vi "CreateChannel.vi"(6 "Units":string, 8 "error in (no error)":errorcluster, 9 "ChannelName":string, 10 "ChannelID":string, 11 "FPGA reference":refnum<k20>) -> (0 "error out":errorcluster, 3 "9770 API out":refnum<class "9770 API.lvclass">)   [LabVIEW 2017, in "9770 API.lvclass"]
uses:
  <vilib>/addons/InsightCM/Devices/Shared/Emsa/Emsa9770API/9770 API.lvclass
  <vilib>/addons/InsightCM/Devices/Shared/Emsa/Emsa9770API/controls/FPGATypeDef.ctl
  <vilib>/addons/InsightCM/Devices/Shared/Emsa/Emsa9770API/9770 API.lvclass/9770 API.ctl
  <vilib>/rvi/interface/common/niFpgaWaitOnOcc.vi
  <vilib>/Utility/error.llb/Error Cluster From Error Code.vi
  <vilib>/rvi/interface/nirviMethod/nirviMethod.xnode
  <vilib>/FPGAPlugInAG/Dynamic/niLvFpga_ConfigureFifo_Dynamic.vi
  <vilib>/rvi/errors/niLvFpgaMergeErrorWithErrorCode.vi
  <vilib>/FPGAPlugInAG/Dynamic/niLvFpga_StartFifo_Dynamic.vi
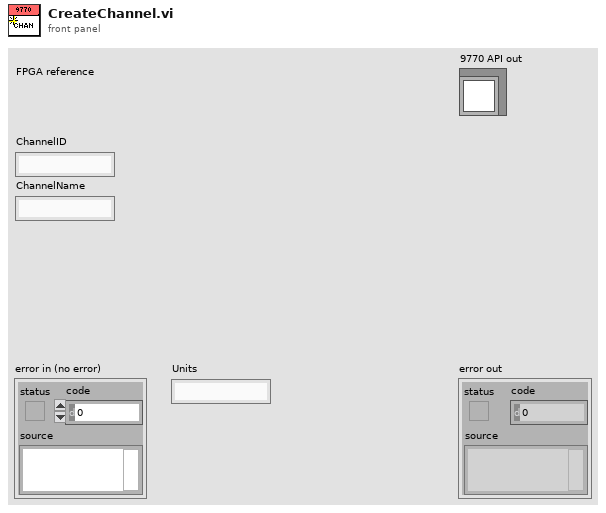
[diagram p1: front panel]
types:
  T1 = typedef "9770 API.lvclass/FPGATypeDef.ctl" = refnum<k20>
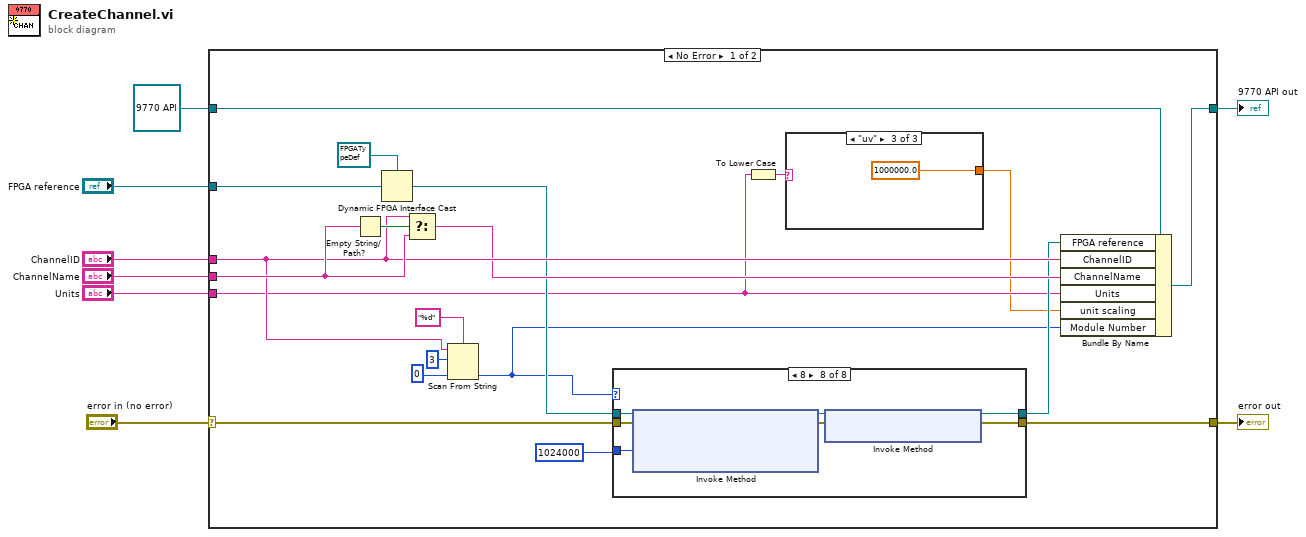
[diagram p0: block diagram]
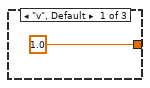
[diagram p2: hidden frame]
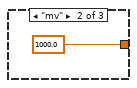
[diagram p3: hidden frame]
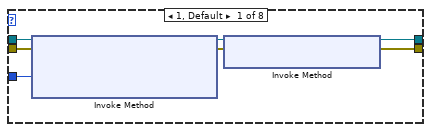
[diagram p4: hidden frame]
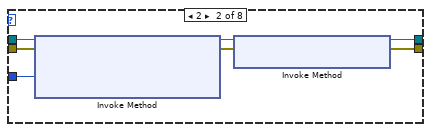
[diagram p5: hidden frame]
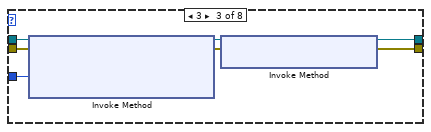
[diagram p6: hidden frame]
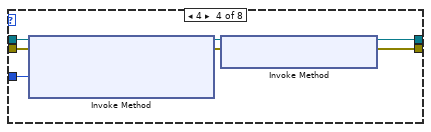
[diagram p7: hidden frame]
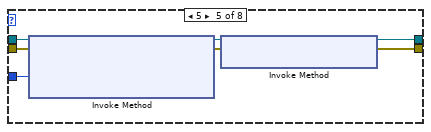
[diagram p8: hidden frame]
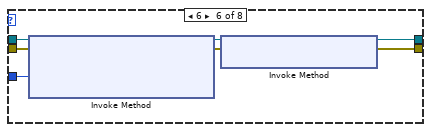
[diagram p9: hidden frame]
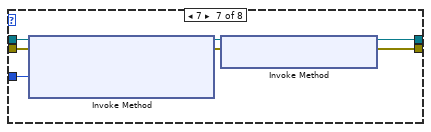
[diagram p10: hidden frame]
diagram:
  n1 = case shown="No Error" "error in (no error)" {
    selector: "error in (no error)" -> [w16 w89]
    tunnel: [w15 w89] -> w7
    tunnel: [w27 w88] -> w5
    tunnel: refnum<class "9770 API.lvclass"> refnum ("9770 API in") -> [w28 w88]
    tunnel: "ChannelID" -> [w21 _]
    tunnel: "ChannelName" -> [w22 _]
    tunnel: "Units" -> [w10 _]
    tunnel: "FPGA reference" -> [w19 _]
    frame No Error {
      n2 = Empty String/Path?(string/path=w22) -> (empty?=w23:bool)
      n3 = Dynamic FPGA Interface Cast(Session In=T1 refnum ("FPGA reference"), Type=w19) -> (Session Out=w14:T1)
      n4 = Select(t=w21, s=w23, f=w22) -> (s? t:f=w20:string)
      n5 = Scan From String(format string="%d", input string=w21, initial scan location=u32 3, default 1=u32 0) -> (output 1=w12:u32)  [unwired: 1 in, 3 out]
      n6 = case shown="8" w12 {
        tunnel: [w36 w42 w50 w57 w64 w71 w78 w85] -> w13
        tunnel: [w35 w43 w49 w56 w63 w70 w77 w84] -> w15
        tunnel: u32 1024000 ("Requested Depth") -> [w32 w39 w46 w53 w60 w67 w74 w81]
        tunnel: w14 -> [w34 w41 w48 w55 w62 w69 w76 w83]
        tunnel: w16 -> [w33 w40 w47 w54 w61 w68 w75 w82]
        frame 1, Default {
          n7 = xnode "Invoke Method"("FPGA VI Reference In"=w34, "error in"=w33, "Requested Depth"=w32) -> ("FPGA VI Reference Out"=w37:T1, "error out"=w38:errorcluster)  [unwired: 1 out]
          n8 = xnode "Invoke Method"("FPGA VI Reference In"=w37, "error in"=w38) -> ("FPGA VI Reference Out"=w36:T1, "error out"=w35:errorcluster)
        }
        frame 2 {
          n9 = xnode "Invoke Method"("FPGA VI Reference In"=w41, "error in"=w40, "Requested Depth"=w39) -> ("FPGA VI Reference Out"=w44:T1, "error out"=w45:errorcluster)  [unwired: 1 out]
          n10 = xnode "Invoke Method"("FPGA VI Reference In"=w44, "error in"=w45) -> ("FPGA VI Reference Out"=w42:T1, "error out"=w43:errorcluster)
        }
        frame 3 {
          n11 = xnode "Invoke Method"("FPGA VI Reference In"=w48, "error in"=w47, "Requested Depth"=w46) -> ("FPGA VI Reference Out"=w52:T1, "error out"=w51:errorcluster)  [unwired: 1 out]
          n12 = xnode "Invoke Method"("FPGA VI Reference In"=w52, "error in"=w51) -> ("FPGA VI Reference Out"=w50:T1, "error out"=w49:errorcluster)
        }
        frame 4 {
          n13 = xnode "Invoke Method"("FPGA VI Reference In"=w55, "error in"=w54, "Requested Depth"=w53) -> ("FPGA VI Reference Out"=w58:T1, "error out"=w59:errorcluster)  [unwired: 1 out]
          n14 = xnode "Invoke Method"("FPGA VI Reference In"=w58, "error in"=w59) -> ("FPGA VI Reference Out"=w57:T1, "error out"=w56:errorcluster)
        }
        frame 5 {
          n15 = xnode "Invoke Method"("FPGA VI Reference In"=w62, "error in"=w61, "Requested Depth"=w60) -> ("FPGA VI Reference Out"=w65:T1, "error out"=w66:errorcluster)  [unwired: 1 out]
          n16 = xnode "Invoke Method"("FPGA VI Reference In"=w65, "error in"=w66) -> ("FPGA VI Reference Out"=w64:T1, "error out"=w63:errorcluster)
        }
        frame 6 {
          n17 = xnode "Invoke Method"("FPGA VI Reference In"=w69, "error in"=w68, "Requested Depth"=w67) -> ("FPGA VI Reference Out"=w73:T1, "error out"=w72:errorcluster)  [unwired: 1 out]
          n18 = xnode "Invoke Method"("FPGA VI Reference In"=w73, "error in"=w72) -> ("FPGA VI Reference Out"=w71:T1, "error out"=w70:errorcluster)
        }
        frame 7 {
          n19 = xnode "Invoke Method"("FPGA VI Reference In"=w76, "error in"=w75, "Requested Depth"=w74) -> ("FPGA VI Reference Out"=w79:T1, "error out"=w80:errorcluster)  [unwired: 1 out]
          n20 = xnode "Invoke Method"("FPGA VI Reference In"=w79, "error in"=w80) -> ("FPGA VI Reference Out"=w78:T1, "error out"=w77:errorcluster)
        }
        frame 8 {
          n21 = xnode "Invoke Method"("FPGA VI Reference In"=w83, "error in"=w82, "Requested Depth"=w81) -> ("FPGA VI Reference Out"=w87:T1, "error out"=w86:errorcluster)  [unwired: 1 out]
          n22 = xnode "Invoke Method"("FPGA VI Reference In"=w87, "error in"=w86) -> ("FPGA VI Reference Out"=w85:T1, "error out"=w84:errorcluster)
        }
      }
      n23 = To Lower Case(string=w10) -> (all lower case string=w11:string)
      n24 = case shown="\"uv\"" w11 {
        tunnel: [1.0 1000.0 1000000.0] -> w9
        frame "v", Default {
        }
        frame "mv" {
        }
        frame "uv" {
        }
      }
      n25 = Bundle By Name(cluster=w28, "FPGA reference"=w13, "ChannelID"=w21, "ChannelName"=w20, "Units"=w10, "unit scaling"=w9, "Module Number"=w12) -> (w27:refnum<class "9770 API.lvclass">)
    }
    frame Error {
    }
  }
  "error out" <- w7
  "9770 API out" <- w5
